vi "ReadConfigure.vi"(8 "error in (no error)":errorcluster, 11 "section":string caption="段") -> (0 "error out":errorcluster, 3 "Para":string[][](array[string]))   [LabVIEW 2016, in "DGUS.lvlib"]
uses:
  DGUS.lvlib
  <vilib>/Utility/config.llb/Read Key (String).vi
  <vilib>/Utility/config.llb/NI_LVConfig.lvlib
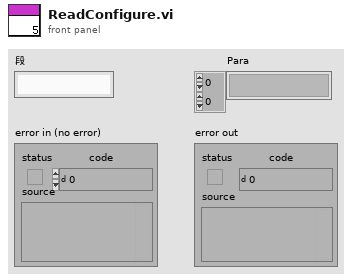
[diagram p1: front panel]
types:
  T1 = typedef "NI_LVConfig.lvlib/Config Data RefNum.ctl" = refnum<k1>
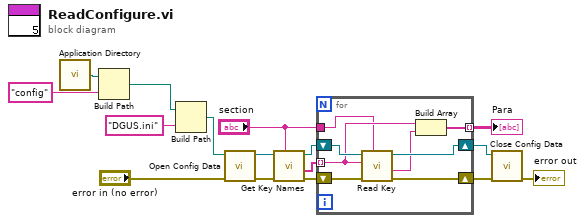
[diagram p0: block diagram]
diagram:
  n1 = call <vilib>:"Application Directory.vi"() -> ("Application Directory"=w14:path)
  n2 = Build Path(base path=w14, name or relative path="config" ("名称或相对路径")) -> (appended path=w12:path)
  n3 = Build Path(base path=w12, name or relative path="DGUS.ini" ("名称或相对路径")) -> (appended path=w10:path)
  n4 = call <vilib>:"Open Config Data.vi"("error in (no error)"="error in (no error)", "configuration file path"=w10) -> ("error out"=w15:errorcluster, "refnum"=w16:T1)  [unwired: 7 in, 1 out]
  n5 = call <vilib>:"Get Key Names.vi"("section"="section", "error in (no error)"=w15, "refnum"=w16) -> ("error out"=w5:errorcluster, "key names"=w6:string[], "refnum out"=w7:T1)  [unwired: 5 in, 1 out]
  n6 = for {
    tunnel: w6 -> [w19] mode=indexing
    shift-right: [w21] -> w4
    shift-left: w7 -> [w24]
    shift-right: [w22] -> w3
    shift-left: w5 -> [w23]
    tunnel: [w18] -> w2 mode=indexing
    tunnel: "section" -> [w17]
    n7 = call-poly <vilib>:"Read Key.vi"("section"=w17, "error in (no error)"=w23, "key"=w19, "refnum"=w24) -> ("error out"=w22:errorcluster, "value"=w20:string, "refnum out"=w21:T1)  [unwired: 4 in, 1 out]
    n8 = Build Array(w19, w20) -> (w18:string[])
  }
  "Para" <- w2
  n9 = call <vilib>:"Close Config Data.vi"("error in (no error)"=w3, "refnum"=w4) -> ("error out"=→"error out":errorcluster)  [unwired: 8 in, 1 out]
